vi "Panel-LAR.vi"() -> ()   [LabVIEW 2009]
uses:
  Instruments/Motor/Controls/MotorStatus.ctl
panel:
  in  "3,AERO-FIE-X,AERO-FIE-Y,AERO-FIE-Z":bool
  out "AERO-FIE-Z":T1
  out "AERO-FIE-X":T1
  out "AERO-FIE-Y":T1
  in  "2,SCHNEE-MS-THETA,SCHNEE-MS-PHI":bool
  out "SCHNEE-MS-PHI":T1
  out "SCHNEE-MS-THETA":T1
  in  "2,SCHNEE-ME-THETA,SCHNEE-ME-PHI":bool
  in  "2,AERO-ME-THETA,AERO-ME-PHI":bool
  out "SCHNEE-ME-PHI":T1
  out "SCHNEE-ME-THETA":T1
  in  "stop":bool
  out "AERO-ME-PHI":T1
  out "AERO-ME-THETA":T1
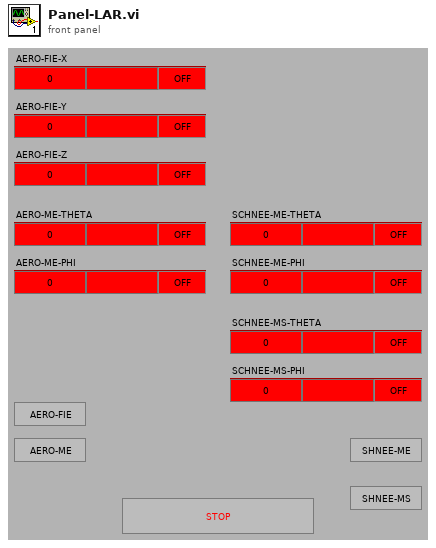
[diagram p1: front panel]
types:
  T1 = typedef "MotorStatus.ctl" = cluster{"Managed?":bool, "Position":i32, "Name":string, "Status":enum16{"OFF", "IDLE", "MOVING", "HOMING"}}
  T2 = enum32{"Invalid", "Standard", "Closed", "Hidden", "Minimized", "Maximized"}
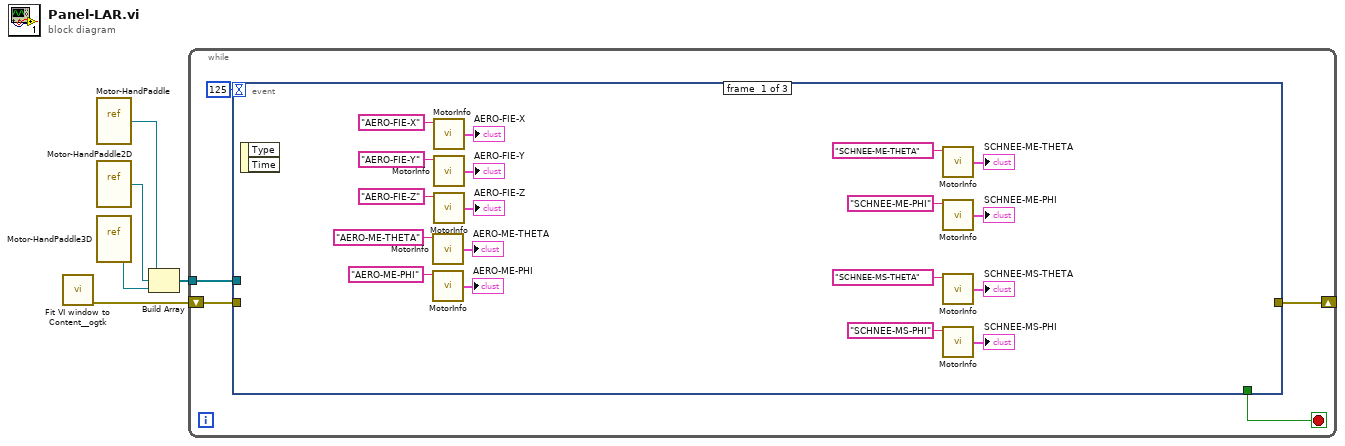
[diagram p0: block diagram]
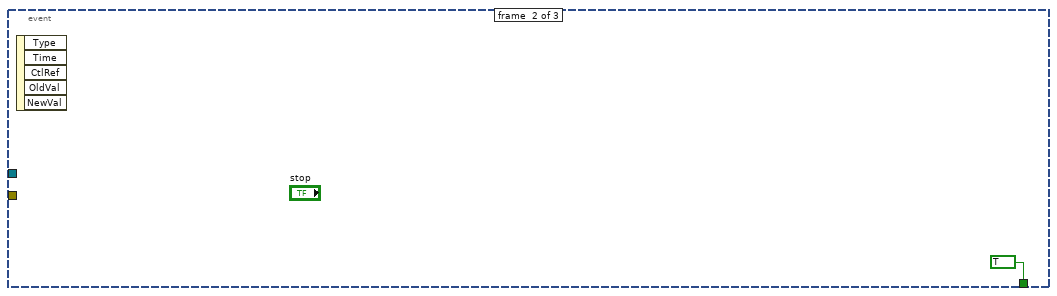
[diagram p2: hidden frame]
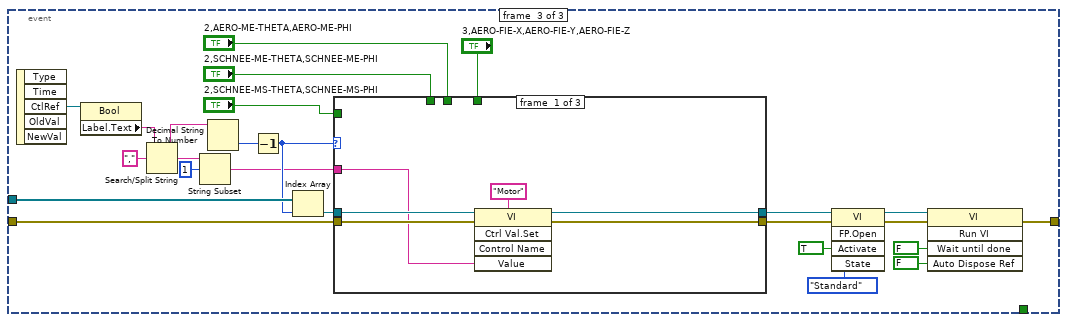
[diagram p3: hidden frame]
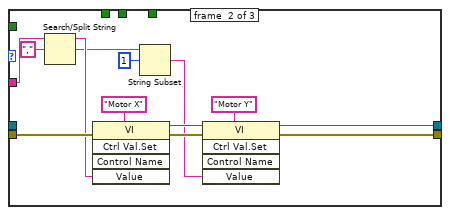
[diagram p4: hidden frame]
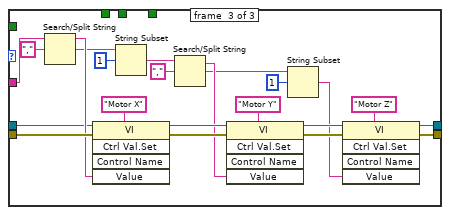
[diagram p5: hidden frame]
diagram:
  n1 = call <userlib>:"Fit VI window to Content__ogtk.vi"() -> ("error out"=w5:errorcluster)  [unwired: 6 in, 1 out]
  n2 = vi-ref "Motor-HandPaddle.vi"() -> (w1:refnum<vi>)
  n3 = vi-ref "Motor-HandPaddle2D.vi"() -> (w4:refnum<vi>)
  n4 = vi-ref "Motor-HandPaddle3D.vi"() -> (w3:refnum<vi>)
  n5 = Build Array(w1, w4, w3) -> (w2:refnum<vi>[])
  n6 = while {
    shift-right: [w8] -> _
    shift-left: w5 -> [w7]
    tunnel: w2 -> [w6]
    stop <- w9 stop-if-true
    n7 = event shown="[2] \"2,AERO-ME-THETA,AERO-ME-PHI\", \"2,SCHNEE-ME-THETA,SCHNEE-ME-PHI\", \"2,SCHNEE-MS-THETA,SCHNEE-MS-PHI\", \"3,AERO-FIE-X,AERO-FIE-Y,AERO-FIE-Z\": Value Change" {
      selector: _ -> [_ _ _]
      dyn-events: _ -> [_ _ _]
      timeout: 125 -> [_ _ _]
      tunnel: [_ TRUE _] -> w9
      tunnel: w7 -> [_ _ w37]
      tunnel: [_ _ w46] -> w8
      tunnel: w6 -> [_ _ w36]
      event #0 {
        n8 = event-data() -> ()  [unwired: 1 in, 2 out]
        n9 = call "MotorInfo.vi"("Motor"="AERO-ME-THETA") -> ("Axis status"=→"AERO-ME-THETA":T1)  [unwired: 1 in, 7 out]
        n10 = call "MotorInfo.vi"("Motor"="AERO-ME-PHI") -> ("Axis status"=→"AERO-ME-PHI":T1)  [unwired: 1 in, 7 out]
        n11 = call "MotorInfo.vi"("Motor"="AERO-FIE-X") -> ("Axis status"=→"AERO-FIE-X":T1)  [unwired: 1 in, 7 out]
        n12 = call "MotorInfo.vi"("Motor"="AERO-FIE-Y") -> ("Axis status"=→"AERO-FIE-Y":T1)  [unwired: 1 in, 7 out]
        n13 = call "MotorInfo.vi"("Motor"="AERO-FIE-Z") -> ("Axis status"=→"AERO-FIE-Z":T1)  [unwired: 1 in, 7 out]
        n14 = call "MotorInfo.vi"("Motor"="SCHNEE-ME-THETA") -> ("Axis status"=→"SCHNEE-ME-THETA":T1)  [unwired: 1 in, 7 out]
        n15 = call "MotorInfo.vi"("Motor"="SCHNEE-ME-PHI") -> ("Axis status"=→"SCHNEE-ME-PHI":T1)  [unwired: 1 in, 7 out]
        n16 = call "MotorInfo.vi"("Motor"="SCHNEE-MS-THETA") -> ("Axis status"=→"SCHNEE-MS-THETA":T1)  [unwired: 1 in, 7 out]
        n17 = call "MotorInfo.vi"("Motor"="SCHNEE-MS-PHI") -> ("Axis status"=→"SCHNEE-MS-PHI":T1)  [unwired: 1 in, 7 out]
      }
      event #1 {
        n18 = event-data() -> ()  [unwired: 1 in, 5 out]
      }
      event #2 {
        n19 = event-data() -> ("CtlRef"=w45:refnum<vi>)  [unwired: 1 in, 4 out]
        n20 = property class="Bool"(reference=w45) -> ("Label.Text"=w43:string)  [unwired: 1 in, 2 out]
        n21 = Search/Split String(string=w43, search string/char (-)=",") -> (substring before match=w33:string, match + rest of string=w42:string)  [unwired: 1 in, 1 out]
        n22 = String Subset(string=w42, offset (0)=1) -> (substring=w30:string)  [unwired: 1 in]
        n23 = Decimal String To Number(string=w33) -> (number=w34:i32)  [unwired: 2 in, 1 out]
        n24 = Decrement(x=w34) -> (x-1=w32:i32)
        n25 = Index Array(array=w36, index=w32) -> (element=w35:refnum<vi>)
        n26 = case shown="2" w32 {
          tunnel: [w60 w72 w81] -> w52
          tunnel: [w59 w67 w84] -> w47
          tunnel: w37 -> [w58 w71 w94]
          tunnel: w35 -> [w57 _ w80]
          tunnel: "2,AERO-ME-THETA,AERO-ME-PHI" -> [_ _ _]
          tunnel: "2,SCHNEE-ME-THETA,SCHNEE-ME-PHI" -> [_ _ _]
          tunnel: "2,SCHNEE-MS-THETA,SCHNEE-MS-PHI" -> [_ _ _]
          tunnel: "3,AERO-FIE-X,AERO-FIE-Y,AERO-FIE-Z" -> [_ _ _]
          tunnel: w30 -> [w55 w61 w73]
          frame #0 {
            n27 = invoke class="VI" method="Ctrl Val.Set"(reference=w57, error in=w58, "Control Name"="Motor", "Value"=w55) -> (reference out=w59:refnum<vi>, error out=w60:errorcluster)  [unwired: 1 in, 3 out]
          }
          frame #1 {
            n28 = Search/Split String(string=w61, search string/char (-)=",") -> (substring before match=w63:string, match + rest of string=w62:string)  [unwired: 1 in, 1 out]
            n29 = invoke class="VI" method="Ctrl Val.Set"(error in=w71, "Control Name"="Motor X", "Value"=w63) -> (reference out=w68:refnum<vi>, error out=w72:errorcluster)  [unwired: 2 in, 3 out]
            n30 = String Subset(string=w62, offset (0)=1) -> (substring=w65:string)  [unwired: 1 in]
            n31 = invoke class="VI" method="Ctrl Val.Set"(reference=w68, "Control Name"="Motor Y", "Value"=w65) -> (reference out=w67:refnum<vi>)  [unwired: 2 in, 4 out]
          }
          frame #2 {
            n32 = Search/Split String(string=w73, search string/char (-)=",") -> (substring before match=w88:string, match + rest of string=w87:string)  [unwired: 1 in, 1 out]
            n33 = invoke class="VI" method="Ctrl Val.Set"(reference=w80, error in=w94, "Control Name"="Motor X", "Value"=w88) -> (reference out=w91:refnum<vi>, error out=w83:errorcluster)  [unwired: 1 in, 3 out]
            n34 = String Subset(string=w87, offset (0)=1) -> (substring=w78:string)  [unwired: 1 in]
            n35 = Search/Split String(string=w78, search string/char (-)=",") -> (substring before match=w77:string, match + rest of string=w75:string)  [unwired: 1 in, 1 out]
            n36 = invoke class="VI" method="Ctrl Val.Set"(reference=w91, error in=w83, "Control Name"="Motor Y", "Value"=w77) -> (reference out=w85:refnum<vi>, error out=w82:errorcluster)  [unwired: 1 in, 3 out]
            n37 = String Subset(string=w75, offset (0)=1) -> (substring=w74:string)  [unwired: 1 in]
            n38 = invoke class="VI" method="Ctrl Val.Set"(reference=w85, error in=w82, "Control Name"="Motor Z", "Value"=w74) -> (reference out=w84:refnum<vi>, error out=w81:errorcluster)  [unwired: 1 in, 3 out]
          }
        }
        n39 = invoke class="VI" method="FP.Open"(reference=w47, error in=w52, "Activate"=TRUE ("Activate?"), "State"=T2."Standard") -> (reference out=w50:refnum<vi>, error out=w51:errorcluster)  [unwired: 1 in, 3 out]
        n40 = invoke class="VI" method="Run VI"(reference=w50, error in=w51, "Wait until done"=FALSE ("Wait Until Done"), "Auto Dispose Ref"=FALSE ("Auto Dispose Reference")) -> (error out=w46:errorcluster)  [unwired: 1 in, 4 out]
      }
    }
  }
